vi "Adjust Splitter.vi"(8 "error in":errorcluster, 9 "Show":bool, 10 "Splitter Info":T1, 11 "Left in":refnum<class "Left.lvclass">) -> (0 "error out":errorcluster, 3 "Left out":refnum<class "Left.lvclass">)   [LabVIEW 2019, in "Left.lvlib" / "Left.lvclass"]
uses:
  Project/Left.lvclass
  C:/Users/Public/Documents/Development/builds/Engine/Engine.lvlibp/Project/Engine.lvclass
  builds/Engine/Engine.lvlibp/Accessors/Read VI_Ref.vi
  builds/Engine/Engine.lvlibp/Project/Engine.lvclass
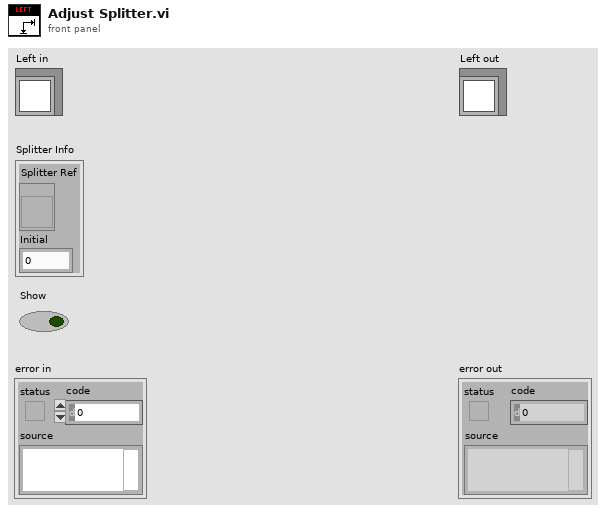
[diagram p1: front panel]
types:
  T1 = cluster{"Splitter Ref":refnum<vi>, "Initial":i32}
  T2 = typedef "LVPointTypeDef.ctl" = cluster{"Horizontal":i16, "Vertical":i16}
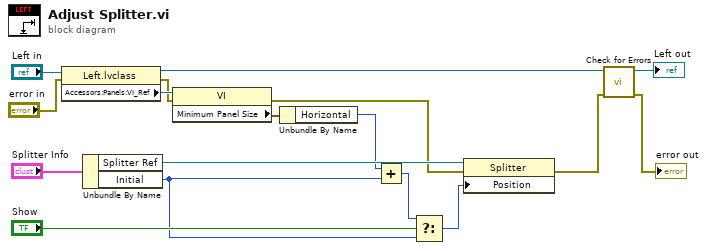
[diagram p0: block diagram]
diagram:
  n1 = property class="Left.lvclass"(reference="Left in", error in="error in") -> (reference out=w4:refnum<class "Left.lvclass">, error out=w6:errorcluster, "Accessors:Panels:VI_Ref"=w14:refnum<vi>)
  n2 = Unbundle By Name("Splitter Info") -> ("Splitter Ref"=w12:refnum<vi>, "Initial"=w9:i32)
  n3 = property class="VI"(reference=w14, error in=w6) -> (error out=w5:errorcluster, "Minimum Panel Size"=w13:T2)  [unwired: 1 out]
  n4 = Unbundle By Name(w13) -> ("Horizontal"=w10:i16)
  n5 = Add(x=w10, y=w9) -> (x+y=w8:i32)
  n6 = Select(t=w8, s="Show", f=w9) -> (s? t:f=w11:i32)
  n7 = property class="Splitter"(reference=w12, error in=w5, "Position"=w11) -> (error out=w2:errorcluster)  [unwired: 1 out]
  n8 = call "Check for Errors.vi"("error in"=w2, "Engine in"=w4) -> ("error out"=→"error out":errorcluster, "Engine out"=→"Left out":refnum<class "Left.lvclass">)  [unwired: 8 in]
